vi "Cgeck LV System.vi"(8 "error in (no error)":errorcluster) -> (0 "error out":errorcluster, 3 "Runtime?":bool)   [LabVIEW 2018]
doc: "returns True if vi using current LabVIEW instance is run time."
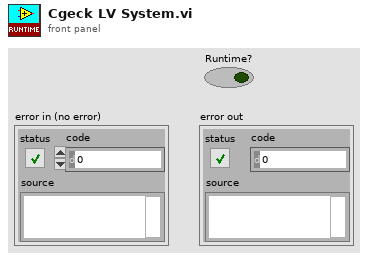
[diagram p1: front panel]
types:
  T1 = enum32{"invalid app kind", "Development System", "Run Time System", "Student Edition", "Embedded LabVIEW", "Evaluation", "Custom"}
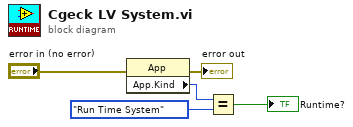
[diagram p0: block diagram]
diagram:
  n1 = property class="App"(error in="error in (no error)") -> (error out=→"error out":errorcluster, "App.Kind"=w1:T1)  [unwired: 1 in, 1 out]
  n2 = Equal?(x=w1, y=T1."Run Time System" ("Application:Kind")) -> (x = y?=→"Runtime?":bool)
